vi "RichToFlatni_measurementlink_discovery_v1_ResolveServiceWithInformationResponse.vi"(5 "OutputClusterType":T1, 11 "InputCluster":T5) -> (3 "OutputCluster":T1)   [LabVIEW 2021, in "ni.measurementlink.discovery.v1.api.lvlib"]
uses:
  ni_measurementlink_discovery_v1_ResolveServiceWithInformationResponse.ctl
  ni_measurementlink_discovery_v1_ServiceLocation.ctl
  ni_measurementlink_discovery_v1_ServiceDescriptor.ctl
  ni_measurementlink_discovery_v1_ServiceDescriptor_AnnotationsEntry.ctl
  ni_measurementlink_discovery_v1_ResolveServiceWithInformationResponse_Flat.ctl
  ni_measurementlink_discovery_v1_ServiceLocation_Flat.ctl
  ni_measurementlink_discovery_v1_ServiceDescriptor_Flat.ctl
  ni_measurementlink_discovery_v1_ServiceDescriptor_AnnotationsEntry_Flat.ctl
  ni.measurementlink.discovery.v1.api.lvlib
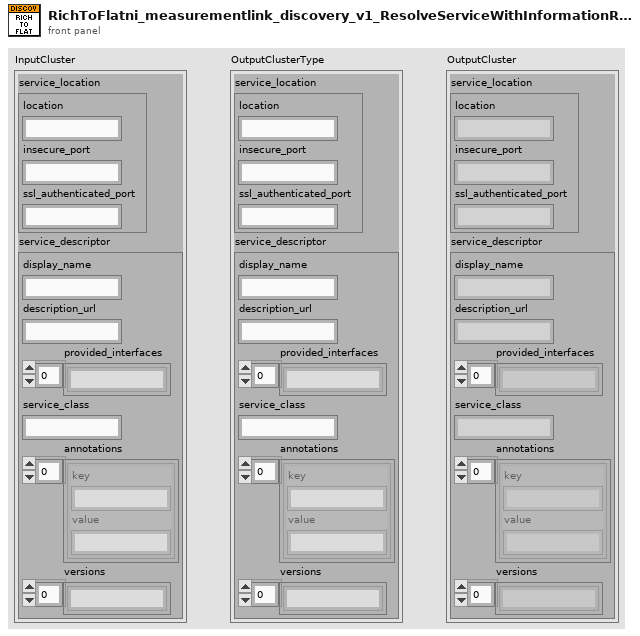
[diagram p1: front panel]
types:
  T1 = typedef "ni.measurementlink.discovery.v1.api.lvlib/ni_measurementlink_discovery_v1_ResolveServiceWithInformationResponse_Flat.ctl" = cluster{"service_location":T2, "service_descriptor":T3}
  T2 = typedef "ni.measurementlink.discovery.v1.api.lvlib/ni_measurementlink_discovery_v1_ServiceLocation_Flat.ctl" = cluster{"location":string, "insecure_port":string, "ssl_authenticated_port":string}
  T3 = typedef "ni.measurementlink.discovery.v1.api.lvlib/ni_measurementlink_discovery_v1_ServiceDescriptor_Flat.ctl" = cluster{"display_name":string, "description_url":string, "provided_interfaces":string[], "service_class":string, "annotations":T4[], "versions":string[]}
  T4 = typedef "ni.measurementlink.discovery.v1.api.lvlib/ni_measurementlink_discovery_v1_ServiceDescriptor_AnnotationsEntry_Flat.ctl" = cluster{"key":string, "value":string}
  T5 = typedef "ni.measurementlink.discovery.v1.api.lvlib/ni_measurementlink_discovery_v1_ResolveServiceWithInformationResponse.ctl" = cluster{"service_location":T6, "service_descriptor":T7}
  T6 = typedef "ni.measurementlink.discovery.v1.api.lvlib/ni_measurementlink_discovery_v1_ServiceLocation.ctl" = cluster{"location":string, "insecure_port":string, "ssl_authenticated_port":string}
  T7 = typedef "ni.measurementlink.discovery.v1.api.lvlib/ni_measurementlink_discovery_v1_ServiceDescriptor.ctl" = cluster{"display_name":string, "description_url":string, "provided_interfaces":string[], "service_class":string, "annotations":T8[], "versions":string[]}
  T8 = typedef "ni.measurementlink.discovery.v1.api.lvlib/ni_measurementlink_discovery_v1_ServiceDescriptor_AnnotationsEntry.ctl" = cluster{"key":string, "value":string}
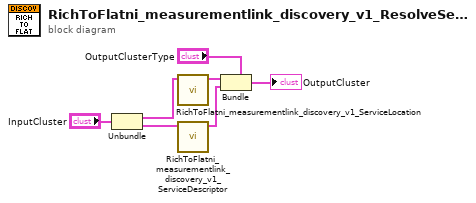
[diagram p0: block diagram]
diagram:
  n1 = Unbundle "Unbundle"("InputCluster") -> ("service_location"=w4:T6, "service_descriptor"=w2:T7)
  n2 = call "RichToFlatni_measurementlink_discovery_v1_ServiceLocation.vi"("InputCluster"=w4) -> ("OutputCluster"=w3:T2)  [unwired: 10 in]
  n3 = call "RichToFlatni_measurementlink_discovery_v1_ServiceDescriptor.vi"("InputCluster"=w2) -> ("OutputCluster"=w1:T3)  [unwired: 10 in]
  n4 = Bundle "Bundle"(cluster="OutputClusterType", "service_location"=w3, "service_descriptor"=w1) -> (→"OutputCluster":T1)
